vi "NewBinnedImageRef.vi"(8 "error in (no error)":errorcluster, 11 "GenericCamera in":refnum<class "GenericCamera.lvclass">) -> (0 "error out":errorcluster, 3 "GenericCamera out":refnum<class "GenericCamera.lvclass">)   [LabVIEW 2013, in "GenericCamera.lvclass"]
uses:
  GenericCamera.lvclass
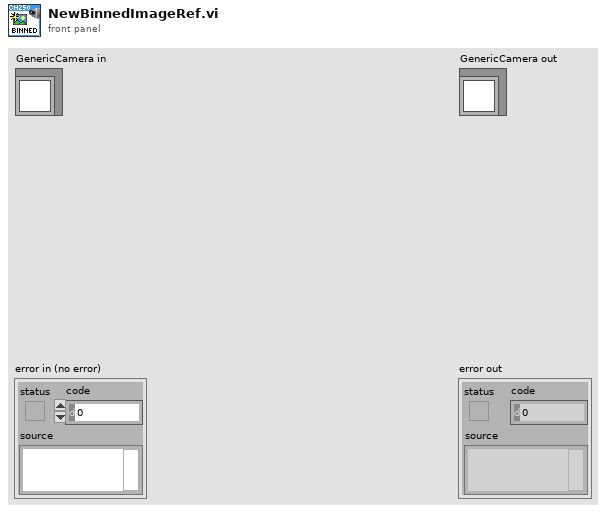
[diagram p1: front panel]
types:
  T1 = typedef "Image Type" = u32
  T2 = typedef "IMAQ Image.ctl" = refnum<image>
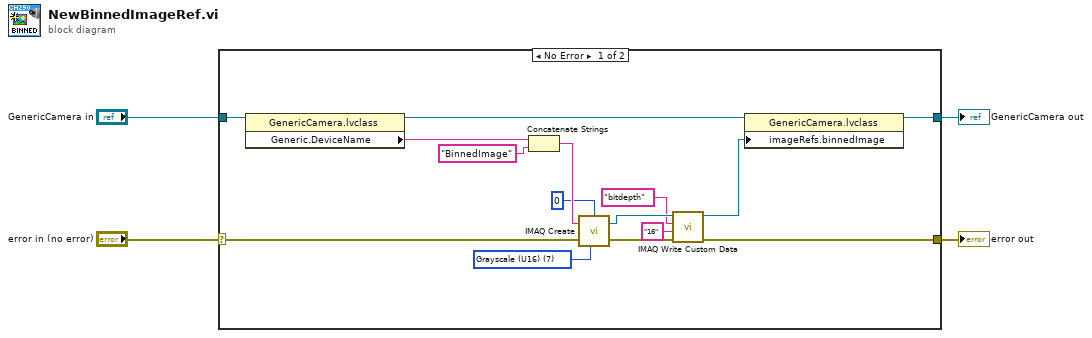
[diagram p0: block diagram]
diagram:
  n1 = case shown="No Error" "error in (no error)" {
    selector: "error in (no error)" -> [w11 w21]
    tunnel: [w10 w21] -> w3
    tunnel: [w9 w20] -> w1
    tunnel: "GenericCamera in" -> [w7 w20]
    frame No Error {
      w13 = T1 7 items=["Grayscale (U8)", "Grayscale (I16)", "Grayscale (SGL)", "Complex (CSG)", "RGB (U32)", "HSL (U32)", "RGB (U64)", "Grayscale (U16)"] ("Image Type")
      n2 = property class="GenericCamera.lvclass"(reference=w7) -> (reference out=w6:refnum<class "GenericCamera.lvclass">, "Generic.DeviceName"=w5:string)  [unwired: 1 in, 1 out]
      n3 = Concatenate Strings(w5, "BinnedImage" ("command or variable name")) -> (w19:string)
      n4 = call "IMAQ Create"("Border Size"=0, "Image Name"=w19, "Image Type"=w13, "error in (no error)"=w11) -> ("New Image"=w15:T2, "error out"=w16:errorcluster)  [unwired: 1 in]
      n5 = call "IMAQ Write Custom Data"("error in (no error)"=w16, "Custom Data In"="16", "Key"="bitdepth", "Image"=w15) -> ("error out"=w10:errorcluster, "Image Out"=w8:T2)  [unwired: 6 in]
      n6 = property class="GenericCamera.lvclass"(reference=w6, "imageRefs.binnedImage"=w8) -> (reference out=w9:refnum<class "GenericCamera.lvclass">)  [unwired: 1 in, 1 out]
    }
    frame Error {
    }
  }
  "error out" <- w3
  "GenericCamera out" <- w1
